vi "Read out RAMP UP.vi"(4 "get more?":bool, 5 "All Channels (T)":bool=TRUE, 7 "Channel":u8, 8 "error in (no error)":errorcluster, 11 "BoardHandle":T2) -> (0 "error out":errorcluster, 1 "Ramp Up constants":T1(array[cluster]), 2 "Ramp up values  (V/s)":i32[](array[numeric]), 3 "BoardHandle out":T2)   [LabVIEW 2020, in "CAEN PSM.lvlib"]
doc: "This function returns Ramp Up rate"
uses:
  CAEN PSM.lvlib
  BoardHandle.ctl
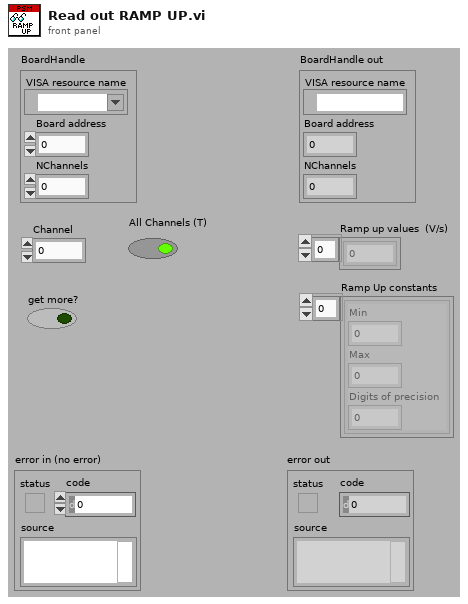
[diagram p1: front panel]
types:
  T1 = cluster{"Min":dbl, "Max":dbl, "Digits of precision":i32}[]
  T2 = typedef "CAEN PSM.lvlib/BoardHandle.ctl" = cluster{"VISA resource name":refnum<visa-resource-name>, "Board address":i8, "NChannels":u8}
  T3 = cluster{"Min":dbl, "Max":dbl, "Digits of precision":i32}
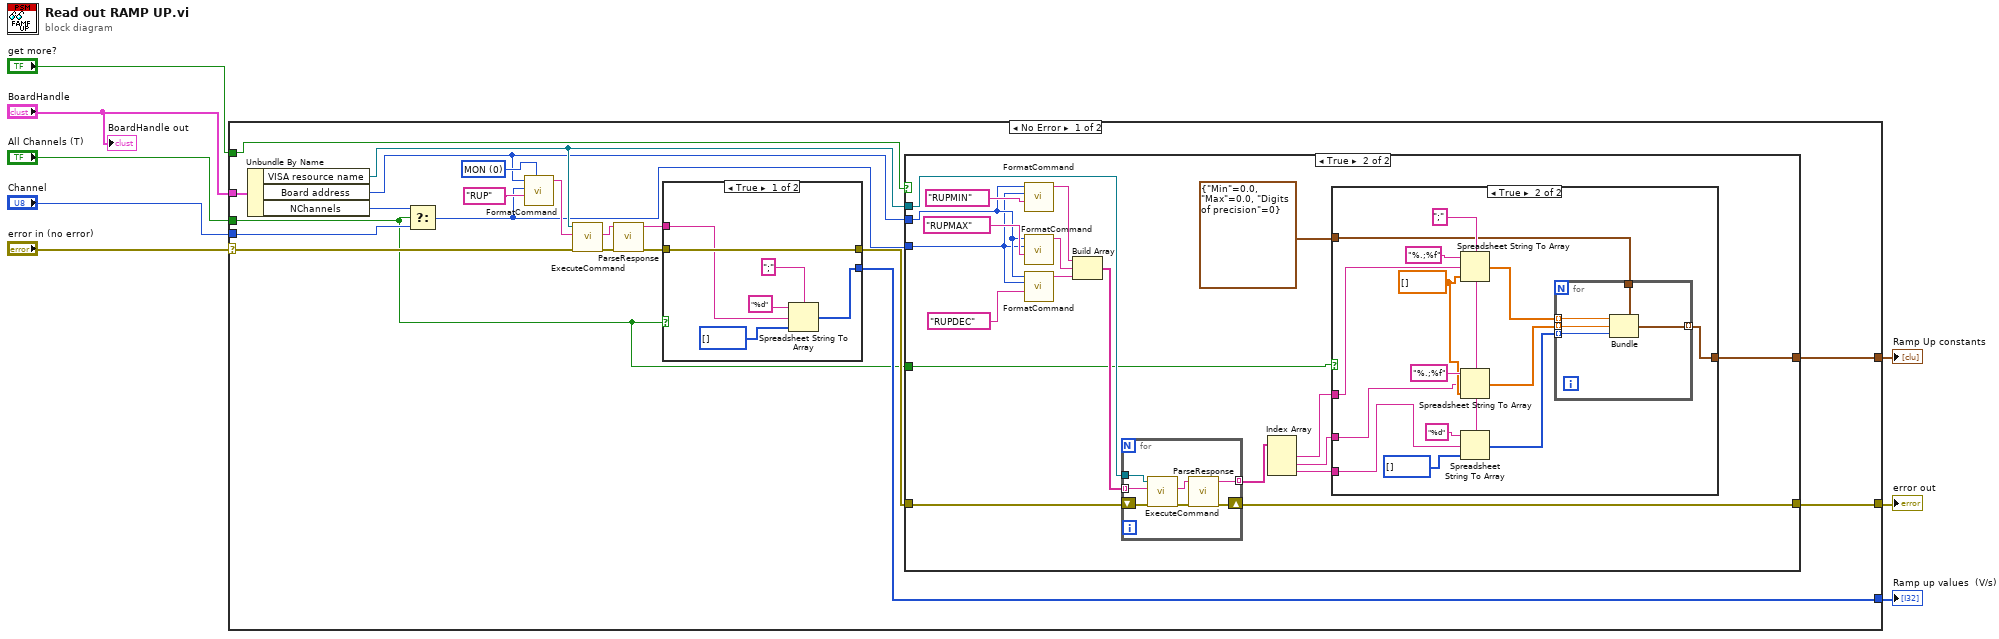
[diagram p0: block diagram]
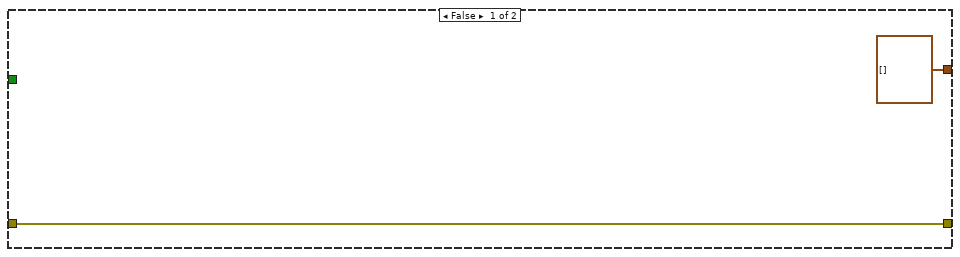
[diagram p2: hidden frame]
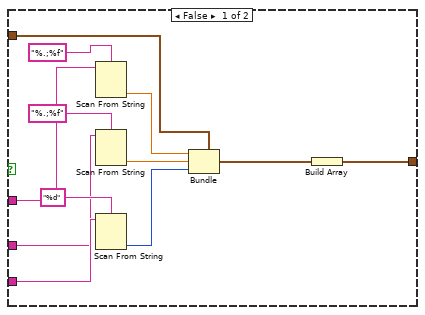
[diagram p3: hidden frame]
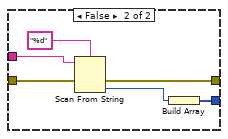
[diagram p4: hidden frame]
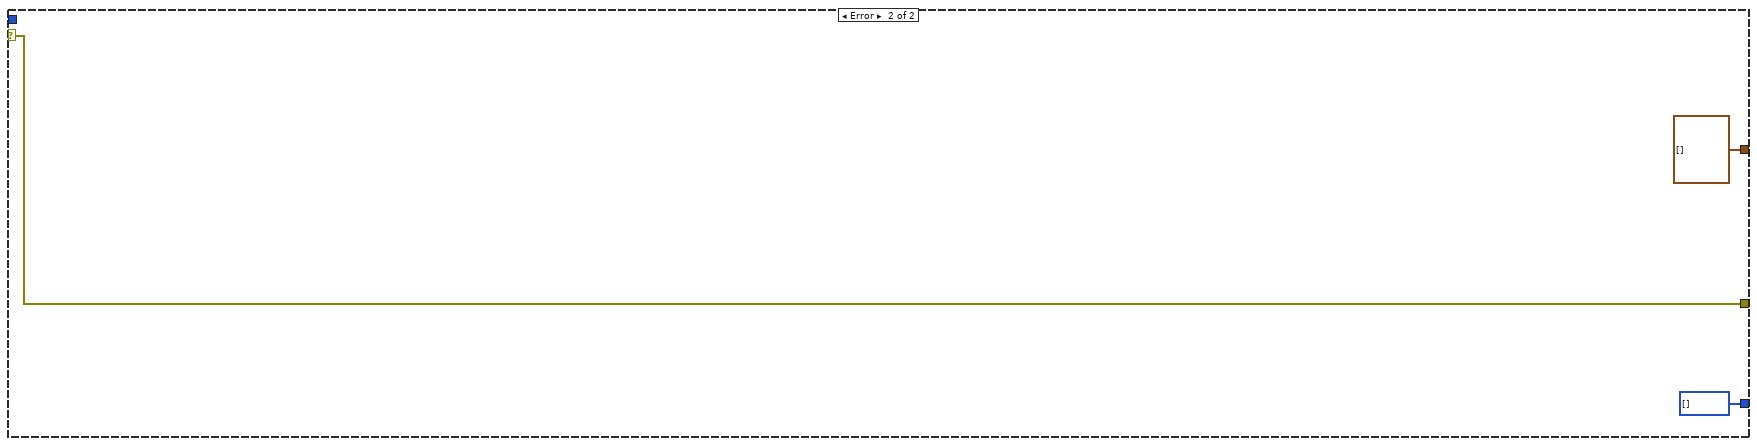
[diagram p5: hidden frame]
diagram:
  n1 = case shown="No Error" "error in (no error)" {
    selector: "error in (no error)" -> [w22 w102]
    tunnel: "All Channels (T)" -> [w9 _]
    tunnel: "Channel" -> [w27 _]
    tunnel: [w12 w102] -> w5
    tunnel: "BoardHandle" -> [w23 _]
    tunnel: [w17 i32[] [] ("Trip value(s) s")] -> w3
    tunnel: [w11 T1 []] -> w2
    tunnel: "get more?" -> [w10 _]
    frame No Error {
      w28 = u8 0 items=["MON", "SET"] ("CMD")
      n2 = Unbundle By Name(w23) -> ("VISA resource name"=w15:refnum<visa-resource-name>, "Board address"=w14:i8, "NChannels"=w20:u8)
      n3 = Select(t=w20, s=w9, f=w27) -> (s? t:f=w13:u8)
      n4 = call "FormatCommand.vi"("CMD (MON)"=w28, "PAR"="RUP", "CH"=w13, "BD (0)"=w14) -> ("cmd"=w26:string)  [unwired: 7 in]
      n5 = call "ExecuteCommand.vi"("error in (no error)"=w22, "Command"=w26, "VISA resource name"=w15) -> ("error out"=w25:errorcluster, "Response"=w24:string)  [unwired: 6 in, 1 out]
      n6 = call "ParseResponse.vi"("error in (no error)"=w25, "Response"=w24) -> ("error out"=w18:errorcluster, "val"=w19:string)  [unwired: 6 in, 2 out]
      n7 = case shown="True" w9 {
        tunnel: w19 -> [w88 w99]
        tunnel: w18 -> [w93 w97]
        tunnel: [w93 w96] -> w16
        tunnel: [w89 w94] -> w17
        frame True {
          n8 = Spreadsheet String To Array(delimiter (Tab)=";", format string="%d", spreadsheet string=w88, array type (2D Dbl)=i32[] []) -> (array=w89:i32[])
        }
        frame False {
          n9 = Scan From String(format string="%d", input string=w99, error in=w97) -> (error out=w96:errorcluster, output 1=w95:i32)  [unwired: 2 in, 2 out]
          n10 = Build Array(w95) -> (w94:i32[])
        }
      }
      n11 = case shown="True" w10 {
        tunnel: w16 -> [w30 w39]
        tunnel: [w30 w38] -> w12
        tunnel: w15 -> [_ w42]
        tunnel: w14 -> [_ w41]
        tunnel: w13 -> [_ w40]
        tunnel: [T1 [] w32] -> w11
        tunnel: w9 -> [_ w31]
        frame False {
        }
        frame True {
          n12 = call "FormatCommand.vi"("PAR"="RUPMIN", "CH"=w40, "BD (0)"=w41) -> ("cmd"=w45:string)  [unwired: 8 in]
          n13 = call "FormatCommand.vi"("PAR"="RUPMAX", "CH"=w40, "BD (0)"=w41) -> ("cmd"=w44:string)  [unwired: 8 in]
          n14 = call "FormatCommand.vi"("PAR"="RUPDEC", "CH"=w40, "BD (0)"=w41) -> ("cmd"=w43:string)  [unwired: 8 in]
          n15 = Build Array(w45, w44, w43) -> (w46:string[])
          n16 = for {
            tunnel: w46 -> [w87] mode=indexing
            tunnel: w42 -> [w86]
            shift-right: [w84] -> w38
            shift-left: w39 -> [w85]
            tunnel: [w81] -> w37 mode=indexing
            n17 = call "ExecuteCommand.vi"("error in (no error)"=w85, "Command"=w87, "VISA resource name"=w86) -> ("error out"=w83:errorcluster, "Response"=w82:string)  [unwired: 6 in, 1 out]
            n18 = call "ParseResponse.vi"("error in (no error)"=w83, "Response"=w82) -> ("error out"=w84:errorcluster, "val"=w81:string)  [unwired: 6 in, 2 out]
          }
          n19 = Index Array(array=w37) -> (element #1=w36:string, element #2=w35:string, element #3=w34:string)  [unwired: 3 in]
          n20 = case shown="True" w31 {
            tunnel: w36 -> [w61 w62]
            tunnel: w35 -> [w56 w63]
            tunnel: w34 -> [w57 w64]
            tunnel: T3 {"Min"=0.0, "Max"=0.0, "Digits of precision"=0} -> [w55 w66]
            tunnel: [w50 w65] -> w32
            frame False {
              n21 = Scan From String(format string="%.;%f", input string=w61) -> (output 1=w54:dbl)  [unwired: 3 in, 3 out]
              n22 = Scan From String(format string="%.;%f", input string=w56) -> (output 1=w53:dbl)  [unwired: 3 in, 3 out]
              n23 = Scan From String(format string="%d", input string=w57) -> (output 1=w52:i32)  [unwired: 3 in, 3 out]
              n24 = Bundle(cluster=w55, "Min"=w54, "Max"=w53, "Digits of precision"=w52) -> (w51:T3)
              n25 = Build Array(w51) -> (w50:T1)
            }
            frame True {
              w70 = dbl[] [] ("array type (2D Dbl)")
              w71 = ";" ("delimiter (Tab)")
              n26 = Spreadsheet String To Array(delimiter (Tab)=w71, format string="%.;%f", spreadsheet string=w62, array type (2D Dbl)=w70) -> (array=w69:dbl[])
              n27 = Spreadsheet String To Array(delimiter (Tab)=w71, format string="%.;%f", spreadsheet string=w63, array type (2D Dbl)=w70) -> (array=w68:dbl[])
              n28 = Spreadsheet String To Array(delimiter (Tab)=w71, format string="%d", spreadsheet string=w64, array type (2D Dbl)=i32[] []) -> (array=w67:i32[])
              n29 = for {
                tunnel: w66 -> [w80]
                tunnel: w69 -> [w79] mode=indexing
                tunnel: w68 -> [w77] mode=indexing
                tunnel: w67 -> [w78] mode=indexing
                tunnel: [w76] -> w65 mode=indexing
                n30 = Bundle(cluster=w80, "Min"=w79, "Max"=w77, "Digits of precision"=w78) -> (w76:T3)
              }
            }
          }
        }
      }
    }
    frame Error {
    }
  }
  "error out" <- w5
  "Ramp up values  (V/s)" <- w3
  "Ramp Up constants" <- w2
  "BoardHandle out" <- "BoardHandle"
